vi "OUT.vi"(8 "error in (no error)":errorcluster, 10 "OUT stat":T2, 11 "refnum in":T1) -> (0 "error out":errorcluster, 3 "refnum out":T1, 4 "question out":string)   [LabVIEW 2018, in "Korad KA3305P.lvlib"]
uses:
  Korad KA3305P.lvlib
  Out stat.ctl
  Reference.ctl
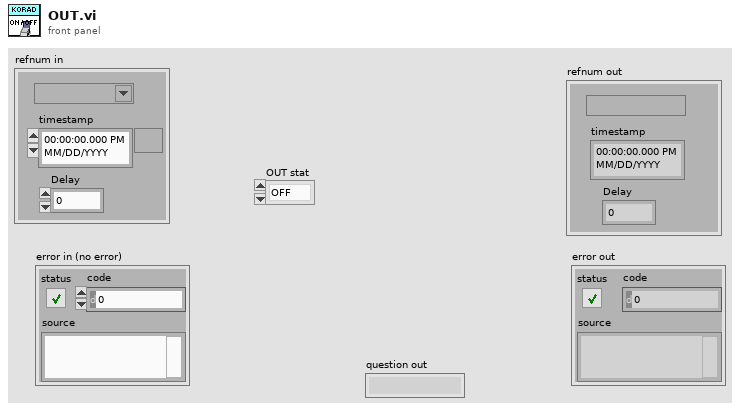
[diagram p1: front panel]
types:
  T1 = typedef "Korad KA3305P.lvlib/Reference.ctl" = cluster{"refnum":refnum<visa-resource-name>, "timestamp":timestamp, "Delay":dbl}
  T2 = typedef "Korad KA3305P.lvlib/Out stat.ctl" = enum16{"OFF", "ON"}
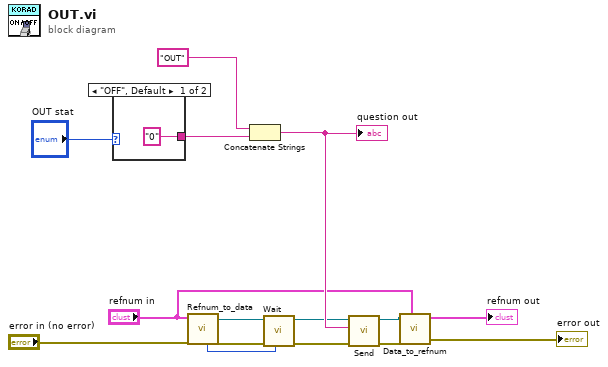
[diagram p0: block diagram]
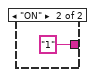
[diagram p2: hidden frame]
diagram:
  n1 = case shown="\"OFF\", Default" "OUT stat" {
    tunnel: ["0" "1"] -> w14
    frame "OFF", Default {
    }
    frame "ON" {
    }
  }
  n2 = call "Refnum_to_data.vi"("error in (no error)"="error in (no error)", "refnum in"="refnum in") -> ("error out"=w7:errorcluster, "DAQ refnum out"=w6:refnum<visa-resource-name>, "delay out"=w1:u32)  [unwired: 7 in]
  n3 = Concatenate Strings("OUT" ("string"), w14) -> (w13:string)
  "question out" <- w13
  n4 = call "Wait.vi"("milliseconds to wait"=w1, "error in (no error)"=w7, "refnum in"=w6) -> ("error out"=w9:errorcluster, "refnum out"=w11:refnum<visa-resource-name>)  [unwired: 7 in]
  n5 = call "Send.vi"("error in (no error)"=w9, "data"=w13, "refnum in"=w11) -> ("error out"=w8:errorcluster, "refnum out"=w3:refnum<visa-resource-name>)  [unwired: 7 in]
  n6 = call "Data_to_refnum.vi"("refnum in"="refnum in", "error in (no error)"=w8, "DAQ refnum in"=w3) -> ("error out"=→"error out":errorcluster, "refnum out"=→"refnum out":T1)  [unwired: 7 in]
